vi "InitBoard.vi"() -> (3 "output array":i32[][](array[numeric]))   [LabVIEW 2018]
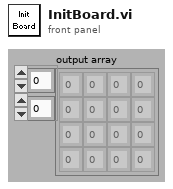
[diagram p1: front panel]
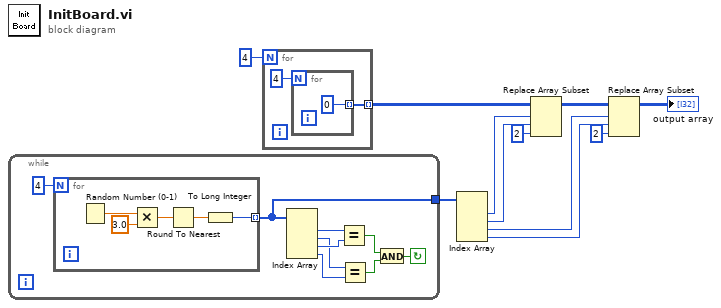
[diagram p0: block diagram]
diagram:
  n1 = while {
    tunnel: [w12] -> w7
    stop <- w13 continue-if-true
    n2 = for {
      N: 4 -> [_]
      tunnel: [w21] -> w12 mode=indexing
      n3 = Random Number (0-1)() -> (number: 0 to 1=w25:dbl)
      n4 = Multiply(x=w25, y=3.0) -> (x*y=w23:dbl)
      n5 = Round To Nearest(number=w23) -> (nearest integer value=w22:dbl)
      n6 = To Long Integer(number=w22) -> (32bit integer=w21:i32)
    }
    n7 = Index Array(array=w12) -> (element #1=w19:i32, element #2=w17:i32, element #3=w18:i32, element #4=w16:i32)  [unwired: 4 in]
    n8 = Equal?(x=w19, y=w18) -> (x = y?=w14:bool)
    n9 = Equal?(x=w17, y=w16) -> (x = y?=w15:bool)
    n10 = And(x=w14, y=w15) -> (x .and. y?=w13:bool)
  }
  n11 = for {
    N: 4 -> [_]
    tunnel: [w26] -> w2 mode=indexing
    n12 = for {
      N: 4 -> [_]
      tunnel: [0 ("Numeric")] -> w26 mode=indexing
    }
  }
  n13 = Index Array(array=w7) -> (element #1=w6:i32, element #2=w5:i32, element #3=w4:i32, element #4=w3:i32)  [unwired: 4 in]
  n14 = Replace Array Subset(array=w2, new element=2 ("index (row)"), index (row)=w6, index (col)=w5) -> (w8:i32[][])
  n15 = Replace Array Subset(array=w8, new element=2 ("index (row)"), index (row)=w4, index (col)=w3) -> (→"output array":i32[][])
